vi "UPRcontroller_v00_basedonlsmv66.vi"() -> ()   [LabVIEW 2015] (continued)
                                tunnel: [w4658 _] -> w4656
                                frame #0 {
                                n1663 = call "waveformparamsv2.vi"("command"="get") -> ("Params out"=w4661:T17)  [unwired: 4 in, 2 out]
                                n1664 = Unbundle By Name(w4661) -> ("DO parameters"=w4662:T20)
                                n1665 = Index Array(array=w4662, index=w4659) -> (element=w4658:T21)
                                }
                                frame #1 {
                                w4676 = 0.0 ("padding value")
                                n1666 = call "2pparameters.vi"("command"="get") -> ("params out"=w4674:T12)  [unwired: 1 in]
                                n1667 = Unbundle By Name(w4674) -> ("srate"=w4672:sgl, "Pel"=w4673:sgl)
                                n1668 = To Double Precision Float(number=w4672) -> (double precision float=w4670:dbl)
                                n1669 = To Double Precision Float(number=w4672) -> (double precision float=w4671:dbl)
                                n1670 = To Double Precision Float(number=w4673) -> (double precision float=w4666:dbl)
                                n1671 = Divide(x=1.0 ("Digital DC (%)"), y=w4666) -> (x/y=w4665:dbl)
                                n1672 = Multiply(x=100.0, y=w4665) -> (x*y=w4664:dbl)
                                n1673 = Divide(x=w4671, y=w4666) -> (x/y=w4669:dbl)
                                n1674 = call "replace DO wf param.vi"("Digital Freq (Hz)"=w4669, "Digital DC (%)"=w4664, "Digital phase"=w4676, "Sampling frequency (Hz)"=w4670, "Digital time offset (s)"=w4676, "index of DO wave"=w4668, "padding value"=w4676, "matlab wave file"=path "LT" ("matlab wave number")) -> ()  [unwired: 3 in]
                                }
                                }
                                }
                                }
                                n1675 = Build Array(w4652) -> (w4651:T20)
                                }
                                }
                                }
                                frame #9 {
                                n1676 = Build Array(w4681, w4680) -> (w4683:bool[])
                                n1677 = Boolean Array To Number(Boolean array=w4683) -> (number=w4682:u32)
                                n1678 = case shown="0" w4682 {
                                tunnel: w4679 -> [_ w4735 _ w4739]
                                tunnel: [_ w4730 _ w4736] -> w4678
                                frame 1 {
                                n1679 = call "2pparameters.vi"("command"="get") -> ("params out"=w4690:T12)  [unwired: 1 in]
                                n1680 = Unbundle By Name(w4690) -> ("wavdet"=w4691:bool, "Pel"=w4693:sgl, "refwfsize"=w4694:dbl, "Pel"=w4692:sgl)
                                n1681 = call "waveformsDObuffer.vi"("command"="get") -> ("DO wf out"=w4686:digitalwaveform[])  [unwired: 1 in]
                                n1682 = case shown="True" w4691 {
                                tunnel: [w4698 w4711] -> w4688
                                tunnel: w4692 -> [w4707 w4726]
                                tunnel: w4693 -> [w4697 w4717]
                                tunnel: w4694 -> [_ w4723]
                                frame False {
                                w4701 = u16 0 items=["unsigned binary", "offset binary", "2's complement"] ("data format (offset binary)")
                                n1683 = Initialize Array(sgl 0.0, w4697) -> (w4704:sgl[])
                                n1684 = Replace Array Subset(array=w4704, new element=sgl 1.0, index=0) -> (w4702:sgl[])
                                n1685 = Reciprocal(x=w4707) -> (1/x=w4708:sgl)
                                n1686 = Bundle By Name("Y"=w4702, "dt"=w4708) -> (w4699:waveform(sgl))  [unwired: 1 in]
                                n1687 = call-poly <vilib>:"Analog to Digital.vi"("data format (offset binary)"=w4701, "compress digital (T)"=TRUE, "full-scale range (pk-pk)"=1.0, "resolution (16 bit)"=1, "analog waveform"=w4699) -> ("digital waveform"=w4698:digitalwaveform)  [unwired: 3 in, 3 out]
                                }
                                frame True {
                                w4714 = u16 0 items=["unsigned binary", "offset binary", "2's complement"] ("data format (offset binary)")
                                n1688 = To Double Precision Float(number=w4717) -> (double precision float=w4724:dbl)
                                n1689 = Initialize Array(sgl 0.0, w4717) -> (w4719:sgl[])
                                n1690 = Divide(x=w4723, y=w4724) -> (x/y=w4721:dbl)
                                n1691 = Round Toward +Infinity(x=w4721) -> (ceil(x): smallest int >= x=w4722:dbl)
                                n1692 = Replace Array Subset(array=w4719, new element=sgl 1.0, index=0) -> (w4716:sgl[])
                                n1693 = for {
                                N: w4722 -> [_]
                                tunnel: w4716 -> [w4728]
                                tunnel: [w4728] -> w4725 mode=concatenating
                                }
                                n1694 = Reciprocal(x=w4726) -> (1/x=w4727:sgl)
                                n1695 = Bundle By Name("Y"=w4725, "dt"=w4727) -> (w4712:waveform(sgl))  [unwired: 1 in]
                                n1696 = call-poly <vilib>:"Analog to Digital.vi"("data format (offset binary)"=w4714, "compress digital (T)"=TRUE, "full-scale range (pk-pk)"=1.0, "resolution (16 bit)"=1, "analog waveform"=w4712) -> ("digital waveform"=w4711:digitalwaveform)  [unwired: 3 in, 3 out]
                                }
                                }
                                n1697 = Build Array (concatenate)(w4686, w4688) -> (w4684:digitalwaveform[])
                                n1698 = call "waveformsDObuffer.vi"("DO wf in"=w4684, "command"="set") -> ()  [unwired: 1 out]
                                }
                                frame 2 {
                                n1699 = call "waveformsDObuffer.vi"("command"="get") -> ("DO wf out"=w4732:digitalwaveform[])  [unwired: 1 in]
                                n1700 = Delete From Array(array=w4732, length=1, index=w4735) -> (deleted portion=w4730:digitalwaveform[], array with subset deleted=w4729:digitalwaveform[])
                                n1701 = call "waveformsDObuffer.vi"("DO wf in"=w4729, "command"="set") -> ()  [unwired: 1 out]
                                }
                                frame 3, Default {
                                }
                                frame 0 {
                                n1702 = local read "Measurement"() -> (w4738:T4)
                                n1703 = To Unsigned Long Integer(number=w4738) -> (unsigned 32bit integer=w4737:u32)
                                n1704 = case shown="5..7" w4737 {
                                tunnel: w4739 -> [_ w4742]
                                tunnel: [_ w4741] -> w4736
                                frame 0..4, Default {
                                }
                                frame 5..7 {
                                n1705 = call "2pparameters.vi"("command"="get") -> ("params out"=w4749:T12)  [unwired: 1 in]
                                n1706 = Unbundle By Name(w4749) -> ("wavdet"=w4750:bool, "Pel"=w4752:sgl, "refwfsize"=w4753:dbl, "srateAODO"=w4751:sgl)
                                n1707 = call "waveformsDObuffer.vi"("command"="get") -> ("DO wf out"=w4743:digitalwaveform[])  [unwired: 1 in]
                                n1708 = Index Array(array=w4743, index=w4742) -> (element=w4744:digitalwaveform)
                                n1709 = case shown="True" w4750 {
                                tunnel: [w4757 w4770] -> w4747
                                tunnel: w4751 -> [w4766 w4785]
                                tunnel: w4752 -> [w4756 w4776]
                                tunnel: w4753 -> [_ w4782]
                                frame False {
                                w4760 = u16 0 items=["unsigned binary", "offset binary", "2's complement"] ("data format (offset binary)")
                                n1710 = Initialize Array(sgl 0.0, w4756) -> (w4763:sgl[])
                                n1711 = Replace Array Subset(array=w4763, new element=sgl 1.0, index=0) -> (w4761:sgl[])
                                n1712 = Reciprocal(x=w4766) -> (1/x=w4767:sgl)
                                n1713 = Bundle By Name("Y"=w4761, "dt"=w4767) -> (w4758:waveform(sgl))  [unwired: 1 in]
                                n1714 = call-poly <vilib>:"Analog to Digital.vi"("data format (offset binary)"=w4760, "compress digital (T)"=TRUE, "full-scale range (pk-pk)"=1.0, "resolution (16 bit)"=1, "analog waveform"=w4758) -> ("digital waveform"=w4757:digitalwaveform)  [unwired: 3 in, 3 out]
                                }
                                frame True {
                                w4773 = u16 0 items=["unsigned binary", "offset binary", "2's complement"] ("data format (offset binary)")
                                n1715 = To Double Precision Float(number=w4776) -> (double precision float=w4783:dbl)
                                n1716 = Initialize Array(sgl 0.0, w4776) -> (w4778:sgl[])
                                n1717 = Divide(x=w4782, y=w4783) -> (x/y=w4780:dbl)
                                n1718 = Round Toward +Infinity(x=w4780) -> (ceil(x): smallest int >= x=w4781:dbl)
                                n1719 = Replace Array Subset(array=w4778, new element=sgl 1.0, index=0) -> (w4775:sgl[])
                                n1720 = for {
                                N: w4781 -> [_]
                                tunnel: w4775 -> [w4787]
                                tunnel: [w4787] -> w4784 mode=concatenating
                                }
                                n1721 = Reciprocal(x=w4785) -> (1/x=w4786:sgl)
                                n1722 = Bundle By Name("Y"=w4784, "dt"=w4786) -> (w4771:waveform(sgl))  [unwired: 1 in]
                                n1723 = call-poly <vilib>:"Analog to Digital.vi"("data format (offset binary)"=w4773, "compress digital (T)"=TRUE, "full-scale range (pk-pk)"=1.0, "resolution (16 bit)"=1, "analog waveform"=w4771) -> ("digital waveform"=w4770:digitalwaveform)  [unwired: 3 in, 3 out]
                                }
                                }
                                n1724 = Build Array(w4744) -> (w4741:digitalwaveform[])
                                n1725 = Replace Array Subset(array=w4743, new element=w4747, index=w4742) -> (w4740:digitalwaveform[])
                                n1726 = call "waveformsDObuffer.vi"("DO wf in"=w4740, "command"="set") -> ()  [unwired: 1 out]
                                }
                                }
                                }
                                }
                                }
                                frame #10 {
                                # "Source of crashing?"
                                n1727 = local read "Meastab"() -> (w4801:enum32{"X-Y Image", "Linescan", "Timetrace"})
                                n1728 = property on="refwf" class="Ring (strict)"() -> ("RingText.Text"=w4798:string)  [unwired: 2 in, 2 out]
                                n1729 = case shown="\"Timetrace\"" w4801 {
                                tunnel: [w4803 w4804] -> w4802
                                frame "X-Y Image", Default {
                                n1730 = local read "Sampling rate"() -> (w4803:dbl)
                                }
                                frame "Timetrace" {
                                n1731 = local read "srateAODOtt"() -> (w4804:dbl)
                                }
                                }
                                n1732 = call "waveformsAObuffer.vi"("command"="get") -> ("AO wf out"=w4791:waveform(dbl)[])  [unwired: 1 in]
                                n1733 = local read "wavdet"() -> (w4799:bool)
                                n1734 = call "waveformsDObuffer.vi"("command"="get") -> ("DO wf out"=w4795:digitalwaveform[])  [unwired: 1 in]
                                n1735 = call "correctwaveformsizetemp.vi"("new sampling frequency (Hz)"=w4802, "start"=TRUE, "reference waveforms to"=w4798, "Analog waveforms in"=w4791, "stop"=FALSE, "Digital waveforms in"=w4795) -> ("analog wf out"=w4797:waveform(dbl)[], "Digital wf out"=w4790:digitalwaveform[], "measpoints"=w4800:i32)
                                n1736 = call "waveformsDObuffer.vi"("DO wf in"=w4790, "command"="set") -> ()  [unwired: 1 out]
                                n1737 = call "waveformsAObuffer.vi"("AO wf in"=w4797, "command"="set") -> ()  [unwired: 1 out]
                                n1738 = case shown="True" w4799 {
                                tunnel: w4800 -> [_ w4807]
                                tunnel: w4790 -> [_ w4805]
                                frame False {
                                }
                                frame True {
                                n1739 = local write "# of frames"(w4807) -> ()
                                n1740 = call "GetNumCamFramesv2.vi"("Digital Waveform Graph"=w4805) -> ("Numeric"=w4806:i32)  [unwired: 10 in]
                                n1741 = local write "Total Camera Frames"(w4806) -> ()
                                }
                                }
                                }
                                }
                              }
                              frame #7 {
                                # "Disabled for conversion to 64 bit"
                                # "lifetime related stuff"
                                n1742 = disable-structure shown="Disabled" {
                                frame Disabled {
                                n1743 = local read "Measurement"() -> (w4809:T4)
                                n1744 = case shown="\"Lifetime (scan)\"" w4809 {
                                frame "X-Y-t movie", Default {
                                }
                                frame "Lifetime (scan)" {
                                # "total acquisition time"
                                n1745 = call "2pparameters.vi"("command"="get") -> ("params out"=w4817:T12)  [unwired: 1 in]
                                n1746 = Unbundle By Name(w4817) -> ("measpoints"=w4811:i32, "srateAODO"=w4832:sgl)
                                n1747 = Divide(x=w4811, y=w4832) -> (x/y=w4810:sgl)
                                n1748 = local read "min phot"() -> (w4827:u32)
                                n1749 = local read "expected c/s"() -> (w4828:dbl)
                                n1750 = Multiply(x=w4810, y=1000.0) -> (x*y=w4820:dbl)
                                n1751 = local read "Ch1 ZeroX"() -> (w4825:i32)
                                n1752 = local read "truncate"() -> (w4826:u32)
                                n1753 = To Long Integer(number=w4820) -> (32bit integer=w4829:i32)
                                n1754 = To Long Integer(number=w4828) -> (32bit integer=w4830:i32)
                                n1755 = local read "Number of Bins"() -> (w4821:u32)
                                n1756 = local read "Ch1 Level"() -> (w4823:i32)
                                n1757 = local read "Ch0 ZeroX"() -> (w4824:i32)
                                n1758 = local write "Acquisition time"(w4829) -> ()
                                n1759 = local read "Ch0 Level"() -> (w4822:i32)
                                n1760 = call "lifetimeparameters.vi"("command"="get") -> ("Params out"=w4815:T22)  [unwired: 1 in]
                                n1761 = Add(x=100, y=w4829) -> (x+y=w4819:i32)
                                n1762 = Bundle By Name(cluster=w4815, "acq time"=w4819, "acq rate"=w4830, "# bins"=w4821, "Ch0 Level"=w4822, "Ch1 Level"=w4823, "Ch0 ZeroX"=w4824, "Ch1 ZeroX"=w4825, "min photons"=w4827, "truncate"=w4826) -> (w4814:T22)
                                n1763 = local write "Acquisition rate"(w4830) -> ()
                                n1764 = call "lifetimeparameters.vi"("Params in"=w4814, "command"="set") -> ()  [unwired: 1 out]
                                }
                                }
                                }
                                frame Enabled {
                                }
                                }
                                n1765 = local write "64bit disabled"(TRUE ("64bit disabled")) -> ()
                              }
                              frame #8 {
                                # "setting timeout and sample mode"
                                n1766 = call "2pparameters.vi"("command"="get") -> ("params out"=w4843:T12)  [unwired: 1 in]
                                n1767 = Unbundle By Name(w4843) -> ("refreshbuffer"=w4841:i32, "srate"=w4842:sgl)
                                n1768 = local read "wavdet"() -> (w4833:bool)
                                n1769 = To Double Precision Float(number=w4842) -> (double precision float=w4845:dbl)
                                n1770 = To Double Precision Float(number=w4841) -> (double precision float=w4836:dbl)
                                n1771 = case shown="False" w4833 {
                                tunnel: [w4850 w4851] -> w4835
                                frame False {
                                w4850 = 10123 items=["Finite Samples"=10178, "Continuous Samples"=10123, "Hardware Timed Single Point"=12522] ("sample mode")
                                }
                                frame True {
                                w4851 = 10123 items=["Finite Samples"=10178, "Continuous Samples"=10123, "Hardware Timed Single Point"=12522] ("sample mode")
                                }
                                }
                                n1772 = Divide(x=w4836, y=w4845) -> (x/y=w4849:dbl)
                                n1773 = Multiply(x=w4849, y=2.0) -> (x*y=w4846:dbl)
                                n1774 = Max & Min(x=w4846, y=10.0) -> (max(x,y)=w4837:dbl)  [unwired: 1 out]
                                n1775 = call "2pparameters.vi"("command"="get") -> ("params out"=w4840:T12)  [unwired: 1 in]
                                n1776 = Bundle By Name(cluster=w4840, "timeout"=w4837, "sample mode"=w4835) -> (w4838:T12)
                                n1777 = call "2pparameters.vi"("Params in"=w4838, "command"="set") -> ()  [unwired: 1 out]
                              }
                            }
                          }
                          frame #1 {
                            # "waveform prepped in prep AO img"
                            # "Disabled for conversion to 64 bit"
                            # "start preparing the tasks"
                            n1778 = call "prepAO_img.vi"() -> ("Terminal Name with Device Prefix"=w4853:tag)
                            n1779 = call "prepDO_img.vi"() -> ()  [unwired: 2 in]
                            n1780 = call "prepAI_img.vi"("triggersource"=w4853) -> ()  [unwired: 2 in]
                            n1781 = call "prepCI_img.vi"("ArmStart.DigEdge.Src"=w4853) -> ()  [unwired: 1 in]
                            n1782 = disable-structure shown="Disabled" {
                              frame Disabled {
                                n1783 = local read "Measurement"() -> (w4854:T4)
                                n1784 = case shown="\"Lifetime (contour)\"" w4854 {
                                frame "X-Y-t movie", Default {
                                }
                                frame "Lifetime (contour)" {
                                n1785 = stacked-sequence {
                                frame #0 {
                                n1786 = call "PH-temp.vi"("String"="clear" ("command")) -> ()  [unwired: 2 in, 2 out]
                                n1787 = call "PH-temp-raw.vi"("command"="empty") -> ()  [unwired: 1 in, 1 out]
                                }
                                frame #1 {
                                n1788 = call "calib.vi"() -> ()  [unwired: 1 in]
                                }
                                frame #2 {
                                n1789 = call "setup.vi"() -> ()  [unwired: 1 in]
                                }
                                }
                                }
                                }
                              }
                              frame Enabled {
                              }
                            }
                            n1790 = local write "64bit disabled"(TRUE ("64bit disabled")) -> ()
                          }
                          frame #2 {
                            # "prepares files for saving"
                            n1791 = local read "save\ndata"() -> (w4857:bool)
                            n1792 = case shown="True" w4857 {
                              tunnel: w4858 -> [_ w4862]
                              frame False {
                              }
                              frame True {
                                n1793 = local read "filename prefix"() -> (w4860:string)
                                n1794 = local read "data dir"() -> (w4861:path)
                                n1795 = call "preparebinaryfiles.vi"("filename prefix"=w4860, "data dir"=w4861, "timestamp"=w4862) -> ("full-filename"=w4859:string)  [unwired: 1 in]
                                n1796 = local write "full-filename"(w4859) -> ()
                              }
                            }
                            n1797 = call "preptempbuffers_tt.vi"() -> ()  [unwired: 12 in]
                          }
                          frame #3 {
                            n1798 = local read "wavdet"() -> (w4863:bool)
                            n1799 = case shown="False" w4863 {
                              frame False {
                                n1800 = disable-structure shown="Disabled" {
                                frame Disabled {
                                n1801 = call "2pparameters.vi"("command"="get") -> ("params out"=w4866:T12)  [unwired: 1 in]
                                n1802 = Unbundle By Name(w4866) -> ("autoshutter"=w4867:bool, "aAS"=w4864:u32[])
                                n1803 = case shown="True" w4867 {
                                tunnel: w4864 -> [_ w4868]
                                frame False {
                                }
                                frame True {
                                n1804 = call "shuttercontrol_multi.vi"("Autoshutter Chans"=w4868, "command"="open") -> ()  [unwired: 1 in, 1 out]
                                }
                                }
                                }
                                frame Enabled {
                                }
                                }
                              }
                              frame True {
                              }
                            }
                          }
                          frame #4 {
                            # "start trigger comes from AO, so  start everything and then start AO"
                            n1805 = flat-sequence {
                              frame #0 {
                                # "Disabled for conversion to 64 bit"
                                n1806 = disable-structure shown="Disabled" {
                                frame Disabled {
                                n1807 = local read "Measurement"() -> (w4871:T4)
                                n1808 = case shown="\"Lifetime (contour)\"" w4871 {
                                frame "X-Y-t movie", Default {
                                }
                                frame "Lifetime (contour)" {
                                n1809 = call "runLT_img.vi"() -> ()  [unwired: 1 in]
                                }
                                }
                                }
                                frame Enabled {
                                }
                                }
                                n1810 = local write "64bit disabled"(TRUE ("64bit disabled")) -> ()
                              }
                              frame #1 {
                                n1811 = call "runAI_img.vi"() -> ()  [unwired: 12 in]
                                n1812 = call "runCI.vi"() -> ()  [unwired: 12 in]
                                n1813 = call "runDO_img.vi"() -> ()  [unwired: 12 in]
                              }
                              frame #2 {
                                n1814 = call "runAO_img.vi"() -> ()  [unwired: 12 in]
                              }
                            }
                          }
                          frame #5 {
                            # "Disabled for conversion to 64 bit"
                            n1815 = while {
                              i -> [w4897]
                              stop <- w4895 stop-if-true
                              n1816 = local read "Stop"() -> (w4905:bool)
                              n1817 = local read "Exit"() -> (w4904:bool)
                              n1818 = Or(x=w4905, y=w4904) -> (x .or. y?=w4903:bool)
                              n1819 = case shown="False" w4903 {
                                frame False {
                                n1820 = stacked-sequence {
                                frame #0 {
                                n1821 = call "collectAI_tt_V2.vi"() -> ()  [unwired: 4 in]
                                n1822 = call "collectCI_tt.vi"() -> ("size(s)"=w4912:i32)  [unwired: 3 in]
                                n1823 = local write "scol"(w4912) -> ()
                                }
                                frame #1 {
                                n1824 = local read "Live"() -> (w4913:bool)
                                n1825 = case shown="True" w4913 {
                                frame False {
                                }
                                frame True {
                                n1826 = local read "graph1list"() -> (w4920:u16)
                                n1827 = local read "graph2list"() -> (w4919:u16)
                                n1828 = To Unsigned Word Integer(number=w4920) -> (unsigned 16bit integer=w4918:u16)
                                n1829 = To Unsigned Word Integer(number=w4919) -> (unsigned 16bit integer=w4917:u16)
                                n1830 = call "dattotrace.vi"("graph2list"=w4917, "Current Average"=sgl 1.0, "graph1list"=w4918) -> ("trace2array out"=w4915:sgl[], "trace1array out"=w4926:sgl[])
                                n1831 = local read "bin"() -> (w4927:dbl)
                                n1832 = script code="data=reshape(datain,[bin length(datain)./bin]);\ndataout=mean(data,1);\ndata2=reshape(datain2,[bin length(datain2)./bin]);\ndataout2=mean(data2,1);"("bin"=w4927, "datain"=w4926, "datain2"=w4915) -> ("dataout"=w4925:dbl[], "dataout2"=w4914:dbl[])  [unwired: 1 in, 1 out]
                                n1833 = Array Size(array=w4914) -> (size(s)=w4928:i32)
                                n1834 = Divide(x=w4928, y=2) -> (x/y=w4930:dbl)
                                n1835 = Round To Nearest(number=w4930) -> (nearest integer value=w4932:dbl)
                                n1836 = Array Size(array=w4925) -> (size(s)=w4937:i32)
                                n1837 = Delete From Array(array=w4914, length=w4932, index=0) -> (deleted portion=w4923:dbl[], array with subset deleted=w4924:dbl[])
                                n1838 = Divide(x=w4937, y=2) -> (x/y=w4935:dbl)
                                n1839 = Round To Nearest(number=w4935) -> (nearest integer value=w4933:dbl)
                                n1840 = Delete From Array(array=w4925, length=w4933, index=0) -> (deleted portion=w4922:dbl[], array with subset deleted=w4921:dbl[])
                                n1841 = local write "graph2"(w4921) -> ()
                                n1842 = local write "graph1"(w4922) -> ()
                                n1843 = local write "graph3"(w4923) -> ()
                                n1844 = local write "graph4"(w4924) -> ()
                                }
                                }
                                }
                                frame #2 {
                                n1845 = local read "save\ndata"() -> (w4938:bool)
                                n1846 = case shown="True" w4938 {
                                frame False {
                                }
                                frame True {
                                n1847 = call "savebinaryfiles.vi"() -> ()  [unwired: 1 in]
                                }
                                }
                                }
                                }
                                }
                                frame True {
                                }
                              }
                              n1848 = Increment(x=w4897) -> (x+1=w4896:i32)
                              n1849 = local write "points recorded"(w4896) -> ()
                              n1850 = local read "continuous"() -> (w4900:bool)
                              n1851 = case shown="False" w4900 {
                                tunnel: w4896 -> [w4910 _]
                                tunnel: [w4909 FALSE] -> w4898
                                frame False {
                                n1852 = call "2pparameters.vi"("command"="get") -> ("params out"=w4907:T12)  [unwired: 1 in]
                                n1853 = Unbundle By Name(w4907) -> ("tt_cycles"=w4906:i32)
                                n1854 = Greater Or Equal?(x=w4910, y=w4906) -> (x >= y?=w4909:bool)
                                }
                                frame True {
                                }
                              }
                              n1855 = local read "Stop"() -> (w4902:bool)
                              n1856 = local read "Exit"() -> (w4901:bool)
                              n1857 = Or(x=w4902, y=w4901) -> (x .or. y?=w4899:bool)
                              n1858 = Or(x=w4899, y=w4898) -> (x .or. y?=w4895:bool)
                            }
                            n1859 = disable-structure shown="Disabled" {
                              disable-tunnel: w4873 -> [w4874 _]
                              frame Disabled {
                                w4877 = u16 0 items=["Stream to disk", "Post process", "real time process"] ("Ring")
                                n1860 = local read "T3R Data processing"() -> (w4876:u16)
                                n1861 = Equal?(x=w4876, y=w4877) -> (x = y?=w4875:bool)
                                n1862 = local read "save\ndata"() -> (w4879:bool)
                                n1863 = local read "Measurement"() -> (w4880:T4)
                                n1864 = And(x=w4879, y=w4875) -> (x .and. y?=w4878:bool)
                                n1865 = case shown="\"Lifetime (contour)\"" w4880 {
                                tunnel: w4874 -> [_ w4884]
                                tunnel: w4878 -> [_ w4882]
                                frame "X-Y-t movie", Default {
                                }
                                frame "Lifetime (contour)" {
                                n1866 = case shown="True" w4882 {
                                selector: w4882 -> [w4885 w4890]
                                tunnel: w4884 -> [_ w4888]
                                tunnel: [path "" ("appended path") w4891] -> w4883
                                tunnel: [w4885 w4890] -> w4881
                                frame False {
                                }
                                frame True {
                                n1867 = local read "filename prefix"() -> (w4889:string)
                                n1868 = local read "data dir"() -> (w4892:path)
                                n1869 = call "generatedatafilename.vi"("timestamp"=w4888, "filename prefix in"=w4889) -> ("full-filename"=w4887:string)
                                n1870 = Concatenate Strings(w4887, ".lvpt3contour" ("string")) -> (w4894:string)
                                n1871 = Build Path(base path=w4892, name or relative path=w4894) -> (appended path=w4891:path)
                                }
                                }
                                n1872 = call "collectLT_res_v1.vi"("stream?"=w4881, "data file"=w4883) -> ()  [unwired: 2 out]
                                }
                                }
                              }
                              frame Enabled {
                              }
                            }
                            n1873 = local write "64bit disabled"(TRUE ("64bit disabled")) -> ()
                          }
                          frame #6 {
                            # "Disabled for conversion to 64 bit"
                            n1874 = local read "Measurement"() -> (w4941:T4)
                            n1875 = disable-structure shown="Disabled" {
                              disable-tunnel: w4941 -> [w4943 _]
                              disable-tunnel: w4940 -> [w4942 _]
                              frame Disabled {
                                n1876 = case shown="\"Lifetime (contour)\"" w4943 {
                                tunnel: w4942 -> [_ w4944]
                                frame "X-Y-t movie", Default {
                                }
                                frame "Lifetime (contour)" {
                                n1877 = stacked-sequence {
                                tunnel: w4944 -> [_ w4945]
                                frame #0 {
                                n1878 = flat-sequence {
                                frame #0 {
                                n1879 = call "stoperaseLT_img.vi"() -> ()  [unwired: 1 in]
                                }
                                }
                                }
                                frame #1 {
                                w4948 = u16 0 items=["Stream to disk", "Post process", "real time process"] ("Ring")
                                n1880 = local read "T3R Data processing"() -> (w4947:u16)
                                n1881 = local read "save\ndata"() -> (w4950:bool)
                                n1882 = Equal?(x=w4947, y=w4948) -> (x = y?=w4946:bool)
                                n1883 = Not(x=w4946) -> (.not. x?=w4951:bool)
                                n1884 = And(x=w4950, y=w4951) -> (x .and. y?=w4949:bool)
                                n1885 = case shown="True" w4949 {
                                tunnel: w4945 -> [_ w4952]
                                frame False {
                                }
                                frame True {
                                n1886 = local read "filename prefix"() -> (w4953:string)
                                n1887 = local read "data dir"() -> (w4969:path)
                                n1888 = call "2pparameters.vi"("command"="get") -> ("params out"=w4964:T12)  [unwired: 1 in]
                                n1889 = call "generatedatafilename.vi"("timestamp"=w4952, "filename prefix in"=w4953) -> ("full-filename"=w4954:string)
                                n1890 = Unbundle By Name(w4964) -> ("srate"=w4962:sgl, "Pel"=w4961:sgl, "measpoints"=w4959:i32)
                                n1891 = Concatenate Strings(w4954, ".lvpt3contour" ("string")) -> (w4967:string)
                                n1892 = Build Path(base path=w4969, name or relative path=w4967) -> (appended path=w4966:path)
                                n1893 = To Unsigned Long Integer(number=w4962) -> (unsigned 32bit integer=w4963:u32)
                                n1894 = To Unsigned Long Integer(number=w4961) -> (unsigned 32bit integer=w4960:u32)
                                n1895 = To Unsigned Long Integer(number=w4959) -> (unsigned 32bit integer=w4958:u32)
                                n1896 = call "PH-temp-raw.vi"("command"="get") -> ("array out"=w4957:u32[])  [unwired: 1 in]
                                n1897 = Build Array (concatenate)(w4963, w4960, w4958, w4957) -> (w4956:u32[])
                                n1898 = Open/Create/Replace File(file path (use dialog)=w4966, operation (0:open)=T9."replace or create") -> (refnum out=w4973:refnum<file>, error out=w4972:errorcluster)  [unwired: 4 in, 1 out]
                                n1899 = Write to Binary File(file (use dialog)=w4973, data=w4956, error in=w4972, 5:FALSE ("prepend array or string size? (T)")) -> (refnum out=w4970:refnum<file>, error out=w4971:errorcluster)  [unwired: 2 in, 1 out]
                                n1900 = Close File(refnum=w4970, error in=w4971) -> ()  [unwired: 2 out]
                                }
                                }
                                }
                                }
                                }
                                }
                              }
                              frame Enabled {
                              }
                            }
                            n1901 = local write "64bit disabled"(TRUE ("64bit disabled")) -> ()
                          }
                          frame #7 {
                            n1902 = flat-sequence {
                              frame #0 {
                                n1903 = call "reset AO_DO_v3.vi"() -> ()  [unwired: 12 in]
                              }
                              frame #1 {
                                n1904 = call "stoperaseCI.vi"() -> ()  [unwired: 12 in]
                                n1905 = call "stoperaseDO_img.vi"() -> ()  [unwired: 12 in]
                                n1906 = call "stoperaseAO_img.vi"() -> ()  [unwired: 12 in]
                                n1907 = call "stoperaseAI_img.vi"() -> ()  [unwired: 12 in]
                              }
                            }
                          }
                          frame #8 {
                            n1908 = stacked-sequence {
                              tunnel: w4989 -> [w4992 _ _ _ _ _]
                              tunnel: w4986 -> [w4991 _ _ _ _ _]
                              tunnel: w4987 -> [w4990 _ _ _ _ _]
                              tunnel: w4988 -> [_ w5041 _ _ _ _]
                              tunnel: w4984 -> [_ w5040 w5091 w5214 _ _]
                              tunnel: w4985 -> [_ w5039 w5092 w5213 _ _]
                              tunnel: w4983 -> [_ _ _ w5212 _ _]
                              tunnel: w4982 -> [_ _ _ w5211 _ _]
                              tunnel: w4981 -> [_ _ w5094 _ _ _]
                              tunnel: w4980 -> [_ _ w5093 _ _ _]
                              tunnel: w4979 -> [_ _ w5088 _ _ _]
                              tunnel: w4978 -> [_ _ w5089 _ _ _]
                              tunnel: w4977 -> [_ _ _ w5209 _ _]
                              tunnel: w4976 -> [_ _ _ w5208 _ _]
                              frame #0 {
                                n1909 = case shown="True" w4992 {
                                tunnel: w4991 -> [_ w5014]
                                tunnel: w4990 -> [_ w5013]
                                frame True {
                                n1910 = stacked-sequence {
                                seq-local: [w4993 _ _] -> [_ w5005 w5010]
                                frame #0 {
                                n1911 = call "configuration.vi"("command"="get") -> ("config out"=w4999:T14)  [unwired: 2 in, 1 out]
                                n1912 = Unbundle By Name(w4999) -> ("Voltage to Xgalvo"=w4996:i32)
                                n1913 = call "2pparameters.vi"("command"="get") -> ("params out"=w4997:T12)  [unwired: 1 in]
                                n1914 = in-place {
                                in-place-border: w4996 -> [w5004]
                                in-place-border: [w5001] -> w4993
                                n1915 = in-place-cluster #31(w4997) -> ("aAO"=w5003:u32[])
                                n1916 = call "remove channel from active arrayv2.vi"("line array in"=w5003, "line to remove"=w5004) -> ("line array out"=w5002:u32[], "index"=w5001:i32)  [unwired: 1 out]
                                n1917 = in-place-cluster #31("aAO"=w5002) -> (w4994:T12)
                                }
                                n1918 = call "2pparameters.vi"("Params in"=w4994, "command"="set") -> ()  [unwired: 1 out]
                                }
                                frame #1 {
                                n1919 = call "waveformparamsv2.vi"("command"="rem AO", "index"=w5005) -> ()  [unwired: 3 in, 3 out]
                                }
                                frame #2 {
                                n1920 = call "waveformsAObuffer.vi"("command"="get") -> ("AO wf out"=w5011:waveform(dbl)[])  [unwired: 1 in]
                                n1921 = Delete From Array(array=w5011, length=1, index=w5010) -> (array with subset deleted=w5007:waveform(dbl)[])  [unwired: 1 out]
                                n1922 = call "waveformsAObuffer.vi"("AO wf in"=w5007, "command"="set") -> ()  [unwired: 1 out]
                                }
                                }
                                }
                                frame False {
                                n1923 = stacked-sequence {
                                seq-local: [w5015 _ _] -> [_ w5023 w5034]
                                tunnel: w5014 -> [_ w5022 _]
                                tunnel: w5013 -> [_ _ w5033]
                                frame #0 {
                                n1924 = call "configuration.vi"("command"="get") -> ("config out"=w5020:T14)  [unwired: 2 in, 1 out]
                                n1925 = Unbundle By Name(w5020) -> ("Voltage to Xgalvo"=w5016:i32)
                                n1926 = call "2pparameters.vi"("command"="get") -> ("params out"=w5019:T12)  [unwired: 1 in]
                                n1927 = Unbundle By Name(w5019) -> ("aAO"=w5017:u32[])
                                n1928 = Search 1D Array(1D array=w5017, element=w5016) -> (index of element=w5015:i32)  [unwired: 1 in]
                                }
                                frame #1 {
                                n1929 = call "waveformparamsv2.vi"("command"="get") -> ("Params out"=w5026:T17)  [unwired: 4 in, 2 out]
                                n1930 = in-place {
                                in-place-border: w5023 -> [w5030]
                                in-place-border: w5022 -> [w5029]
                                n1931 = in-place-cluster #32(w5026) -> ("AO parameters"=w5031:T18)
                                n1932 = in-place {
                                in-place-border: w5029 -> [w5032]
                                n1933 = in-place-array #33(w5031, w5030) -> ()  [unwired: 1 out]
                                n1934 = in-place-array #33(w5032) -> (w5028:T18)  [unwired: 1 out]
                                }
                                n1935 = in-place-cluster #32("AO parameters"=w5028) -> (w5024:T17)
                                }
                                n1936 = call "waveformparamsv2.vi"("command"="set", "Params in"=w5024) -> ()  [unwired: 3 in, 3 out]
                                }
                                frame #2 {
                                n1937 = call "waveformsAObuffer.vi"("command"="get") -> ("AO wf out"=w5037:waveform(dbl)[])  [unwired: 1 in]
                                n1938 = Replace Array Subset(array=w5037, new element=w5033, index=w5034) -> (w5035:waveform(dbl)[])
                                n1939 = call "waveformsAObuffer.vi"("AO wf in"=w5035, "command"="set") -> ()  [unwired: 1 out]
                                }
                                }
                                }
                                }
                              }
                              frame #1 {
                                n1940 = case shown="True" w5041 {
                                tunnel: w5040 -> [_ w5063]
                                tunnel: w5039 -> [_ w5062]
                                frame True {
                                n1941 = stacked-sequence {
                                seq-local: [w5042 _ _] -> [_ w5054 w5059]
                                frame #0 {
                                n1942 = call "configuration.vi"("command"="get") -> ("config out"=w5048:T14)  [unwired: 2 in, 1 out]
                                n1943 = Unbundle By Name(w5048) -> ("Voltage to Ygalvo"=w5045:i32)
                                n1944 = call "2pparameters.vi"("command"="get") -> ("params out"=w5046:T12)  [unwired: 1 in]
                                n1945 = in-place {
                                in-place-border: w5045 -> [w5053]
                                in-place-border: [w5050] -> w5042
                                n1946 = in-place-cluster #34(w5046) -> ("aAO"=w5052:u32[])
                                n1947 = call "remove channel from active arrayv2.vi"("line array in"=w5052, "line to remove"=w5053) -> ("line array out"=w5051:u32[], "index"=w5050:i32)  [unwired: 1 out]
                                n1948 = in-place-cluster #34("aAO"=w5051) -> (w5043:T12)
                                }
                                n1949 = call "2pparameters.vi"("Params in"=w5043, "command"="set") -> ()  [unwired: 1 out]
                                }
                                frame #1 {
                                n1950 = call "waveformparamsv2.vi"("command"="rem AO", "index"=w5054) -> ()  [unwired: 3 in, 3 out]
                                }
                                frame #2 {
                                n1951 = call "waveformsAObuffer.vi"("command"="get") -> ("AO wf out"=w5060:waveform(dbl)[])  [unwired: 1 in]
                                n1952 = Delete From Array(array=w5060, length=1, index=w5059) -> (array with subset deleted=w5056:waveform(dbl)[])  [unwired: 1 out]
                                n1953 = call "waveformsAObuffer.vi"("AO wf in"=w5056, "command"="set") -> ()  [unwired: 1 out]
                                }
                                }
                                }
                                frame False {
                                n1954 = stacked-sequence {
                                seq-local: [w5064 _ _] -> [_ w5072 w5083]
                                tunnel: w5063 -> [_ w5071 _]
                                tunnel: w5062 -> [_ _ w5082]
                                frame #0 {
                                n1955 = call "configuration.vi"("command"="get") -> ("config out"=w5069:T14)  [unwired: 2 in, 1 out]
                                n1956 = Unbundle By Name(w5069) -> ("Voltage to Ygalvo"=w5065:i32)
                                n1957 = call "2pparameters.vi"("command"="get") -> ("params out"=w5068:T12)  [unwired: 1 in]
                                n1958 = Unbundle By Name(w5068) -> ("aAO"=w5066:u32[])
                                n1959 = Search 1D Array(1D array=w5066, element=w5065) -> (index of element=w5064:i32)  [unwired: 1 in]
                                }
                                frame #1 {
                                n1960 = call "waveformparamsv2.vi"("command"="get") -> ("Params out"=w5075:T17)  [unwired: 4 in, 2 out]
                                n1961 = in-place {
                                in-place-border: w5072 -> [w5079]
                                in-place-border: w5071 -> [w5078]
                                n1962 = in-place-cluster #35(w5075) -> ("AO parameters"=w5080:T18)
                                n1963 = in-place {
                                in-place-border: w5078 -> [w5081]
                                n1964 = in-place-array #36(w5080, w5079) -> ()  [unwired: 1 out]
                                n1965 = in-place-array #36(w5081) -> (w5077:T18)  [unwired: 1 out]
                                }
                                n1966 = in-place-cluster #35("AO parameters"=w5077) -> (w5073:T17)
                                }
                                n1967 = call "waveformparamsv2.vi"("command"="set", "Params in"=w5073) -> ()  [unwired: 3 in, 3 out]
                                }
                                frame #2 {
                                n1968 = call "waveformsAObuffer.vi"("command"="get") -> ("AO wf out"=w5086:waveform(dbl)[])  [unwired: 1 in]
                                n1969 = Replace Array Subset(array=w5086, new element=w5082, index=w5083) -> (w5084:waveform(dbl)[])
                                n1970 = call "waveformsAObuffer.vi"("AO wf in"=w5084, "command"="set") -> ()  [unwired: 1 out]
                                }
                                }
                                }
                                }
                              }
                              frame #2 {
                                n1971 = Build Array(w5094, w5093) -> (w5095:bool[])
                                n1972 = Boolean Array To Number(Boolean array=w5095) -> (number=w5090:u32)
                                n1973 = case shown="0" w5090 {
                                tunnel: w5091 -> [_ _ w5155]
                                tunnel: w5092 -> [_ _ w5154]
                                tunnel: w5088 -> [_ w5125 w5152]
                                tunnel: w5089 -> [_ w5124 w5153]
                                frame 1, Default {
                                n1974 = stacked-sequence {
                                seq-local: [w5098 _ _] -> [_ w5110 w5115]
                                frame #0 {
                                # "Remove autoshutter channel from DO list in 2p parameters"
                                n1975 = call "2pparameters.vi"("command"="get") -> ("params out"=w5097:T12)  [unwired: 1 in]
                                n1976 = Unbundle By Name(w5097) -> ("aAS"=w5096:u32[])
                                n1977 = for {
                                tunnel: [w5104] -> w5098 mode=indexing
                                tunnel: w5096 -> [w5102] mode=indexing
                                shift-right: [w5105] -> w5099
                                shift-left: w5097 -> [w5103]
                                n1978 = in-place {
                                in-place-border: w5102 -> [w5109]
                                in-place-border: [w5106] -> w5104
                                n1979 = in-place-cluster #37(w5103) -> ("aDO"=w5108:u32[])
                                n1980 = call "remove channel from active arrayv2.vi"("line array in"=w5108, "line to remove"=w5109) -> ("line array out"=w5107:u32[], "index"=w5106:i32)  [unwired: 1 out]
                                n1981 = in-place-cluster #37("aDO"=w5107) -> (w5105:T12)
                                }
                                }
                                n1982 = call "2pparameters.vi"("Params in"=w5099, "command"="set") -> ()  [unwired: 1 out]
                                }
                                frame #1 {
                                n1983 = for {
                                tunnel: w5110 -> [w5111] mode=indexing
                                n1984 = call "waveformparamsv2.vi"("command"="rem DO", "index"=w5111) -> ()  [unwired: 3 in, 3 out]
                                }
                                }
                                frame #2 {
                                # "sort so it removes the last elements first\nand does not mess up the order"
                                # "Remove waveforms of autoshutter channels from wave forms DO"
                                n1985 = call "waveformsDObuffer.vi"("command"="get") -> ("DO wf out"=w5118:digitalwaveform[])  [unwired: 1 in]
                                n1986 = Sort 1D Array(array=w5115) -> (sorted array=w5114:i32[])
                                n1987 = Reverse 1D Array(array=w5114) -> (reversed array=w5113:i32[])
                                n1988 = for {
                                tunnel: w5113 -> [w5120] mode=indexing
                                shift-right: [w5121] -> w5116
                                shift-left: w5118 -> [w5123]
                                n1989 = Delete From Array(array=w5123, length=1, index=w5120) -> (array with subset deleted=w5121:digitalwaveform[])  [unwired: 1 out]
                                }
                                n1990 = call "waveformsDObuffer.vi"("DO wf in"=w5116, "command"="set") -> ()  [unwired: 1 out]
                                }
                                }
                                }
                                frame 2 {
                                n1991 = stacked-sequence {
                                tunnel: w5125 -> [_ w5139 _]
                                tunnel: w5124 -> [_ _ w5146]
                                frame #0 {
                                # "add autoshutter channels to digital out"
                                n1992 = disable-structure shown="Disabled" {
                                frame Disabled {
                                n1993 = call "configuration.vi"("command"="get") -> ("config out"=w5131:T14)  [unwired: 2 in, 1 out]
                                n1994 = Unbundle By Name(w5131) -> ()  [unwired: 1 out]
                                }
                                frame Enabled {
                                }
                                }
                                n1995 = call "2pparameters.vi"("command"="get") -> ("params out"=w5127:T12)  [unwired: 1 in]
                                n1996 = Unbundle By Name(w5127) -> ("aAS"=w5126:u32[])
                                n1997 = in-place {
                                in-place-border: w5126 -> [w5133]
                                n1998 = in-place-cluster #38(w5127) -> ("aDO"=w5135:u32[])
                                n1999 = for {
                                shift-right: [w5137] -> w5134
                                shift-left: w5135 -> [w5138]
                                tunnel: w5133 -> [w5136] mode=indexing
                                n2000 = call "add channel to active arrayv2.vi"("line array in"=w5138, "line to add"=w5136) -> ("line array out"=w5137:u32[])  [unwired: 2 out]
                                }
                                n2001 = in-place-cluster #38("aDO"=w5134) -> (w5128:T12)
                                }
                                n2002 = call "2pparameters.vi"("Params in"=w5128, "command"="set") -> ()  [unwired: 1 out]
                                }
                                frame #1 {
                                # "Not sure the correct way to add multiple sets of parameters..."
                                # "add autoshutter waveforms to wf parameters v2"
                                n2003 = disable-structure shown="Disabled" {
                                disable-tunnel: w5139 -> [w5141 _]
                                frame Disabled {
                                n2004 = for {
                                tunnel: w5141 -> [w5142] mode=indexing
                                n2005 = call "waveformparamsv2.vi"("command"="add DO", "add DO"=w5142) -> ()  [unwired: 3 in, 3 out]
                                }
                                }
                                frame Enabled {
                                }
                                }
                                n2006 = call "waveformparamsv2.vi"("command"="add DO", "add DO"=w5139) -> ()  [unwired: 3 in, 3 out]
                                }
                                frame #2 {
                                # "add autoshutter waveforms to wave forms DO"
                                n2007 = call "waveformsDObuffer.vi"("command"="get") -> ("DO wf out"=w5147:digitalwaveform[])  [unwired: 1 in]
                                n2008 = for {
                                tunnel: w5146 -> [w5150] mode=indexing
                                shift-right: [w5149] -> w5144
                                shift-left: w5147 -> [w5151]
                                n2009 = Build Array (concatenate)(w5151, w5150) -> (w5149:digitalwaveform[])
                                }
                                n2010 = call "waveformsDObuffer.vi"("DO wf in"=w5144, "command"="set") -> ()  [unwired: 1 out]
                                }
                                }
                                }
                                frame 0 {
                                n2011 = stacked-sequence {
                                seq-local: [w5157 _ _] -> [_ w5165 w5189]
                                tunnel: w5155 -> [_ _ _]
                                tunnel: w5154 -> [_ _ _]
                                tunnel: w5153 -> [_ _ w5188]
                                tunnel: w5152 -> [_ w5164 _]
                                frame #0 {
                                n2012 = call "2pparameters.vi"("command"="get") -> ("params out"=w5160:T12)  [unwired: 1 in]
                                n2013 = Unbundle By Name(w5160) -> ("aDO"=w5158:u32[], "aAS"=w5156:u32[])
                                n2014 = for {
                                tunnel: w5158 -> [w5163]
                                tunnel: [w5162] -> w5157 mode=indexing
                                tunnel: w5156 -> [w5161] mode=indexing
                                n2015 = Search 1D Array(1D array=w5163, element=w5161) -> (index of element=w5162:i32)  [unwired: 1 in]
                                }
                                }
                                frame #1 {
                                n2016 = call "2pparameters.vi"("command"="get") -> ("params out"=w5168:T12)  [unwired: 1 in]
                                n2017 = Unbundle By Name(w5168) -> ("wavdet"=w5166:bool, "autoshutter"=w5167:bool)
                                n2018 = case shown="True" w5167 {
                                tunnel: w5165 -> [_ w5172]
                                tunnel: w5166 -> [_ w5171]
                                tunnel: w5164 -> [_ w5170]
                                frame False {
                                }
                                frame True {
                                n2019 = case shown="False" w5171 {
                                tunnel: w5172 -> [w5174 _]
                                tunnel: w5170 -> [w5173 _]
                                frame False {
                                # "Replace autoshutter channel DO waveforms with those that were generated from autoshutter."
                                n2020 = call "waveformparamsv2.vi"("command"="get") -> ("Params out"=w5177:T17)  [unwired: 4 in, 2 out]
                                n2021 = in-place {
                                in-place-border: w5174 -> [w5181]
                                in-place-border: w5173 -> [w5179]
                                n2022 = in-place-cluster #39(w5177) -> ("DO parameters"=w5182:T20)
                                n2023 = for {
                                tunnel: w5181 -> [w5185] mode=indexing
                                tunnel: w5179 -> [w5183] mode=indexing
                                shift-right: [w5184] -> w5180
                                shift-left: w5182 -> [w5186]
                                n2024 = in-place {
                                in-place-border: w5183 -> [w5187]
                                n2025 = in-place-array #40(w5186, w5185) -> ()  [unwired: 1 out]
                                n2026 = in-place-array #40(w5187) -> (w5184:T20)  [unwired: 1 out]
                                }
                                }
                                n2027 = in-place-cluster #39("DO parameters"=w5180) -> (w5175:T17)
                                }
                                n2028 = call "waveformparamsv2.vi"("command"="set", "Params in"=w5175) -> ()  [unwired: 3 in, 3 out]
                                }
                                frame True {
                                }
                                }
                                }
                                }
                                }
                                frame #2 {
                                n2029 = call "2pparameters.vi"("command"="get") -> ("params out"=w5192:T12)  [unwired: 1 in]
                                n2030 = Unbundle By Name(w5192) -> ("wavdet"=w5190:bool, "autoshutter"=w5191:bool)
                                n2031 = case shown="True" w5191 {
                                tunnel: w5189 -> [_ w5196]
                                tunnel: w5190 -> [_ w5195]
                                tunnel: w5188 -> [_ w5194]
                                frame False {
                                }
                                frame True {
                                n2032 = case shown="False" w5195 {
                                tunnel: w5196 -> [w5198 _]
                                tunnel: w5194 -> [w5197 _]
                                frame False {
                                # "replace autoshutter channels of waveforms DO with autoshutter waveforms"
                                n2033 = call "waveformsDObuffer.vi"("command"="get") -> ("DO wf out"=w5200:digitalwaveform[])  [unwired: 1 in]
                                n2034 = for {
                                tunnel: w5198 -> [w5204] mode=indexing
                                tunnel: w5197 -> [w5203] mode=indexing
                                shift-right: [w5206] -> w5202
                                shift-left: w5200 -> [w5205]
                                n2035 = Replace Array Subset(array=w5205, new element=w5203, index=w5204) -> (w5206:digitalwaveform[])
                                }
                                n2036 = call "waveformsDObuffer.vi"("DO wf in"=w5202, "command"="set") -> ()  [unwired: 1 out]
                                }
                                frame True {
                                }
                                }
                                }
                                }
                                }
                                }
                                }
                                }
                              }
                              frame #3 {
                                n2037 = Build Array(w5209, w5208) -> (w5210:bool[])
                                n2038 = Boolean Array To Number(Boolean array=w5210) -> (number=w5207:u32)
                                n2039 = case shown="2" w5207 {
                                tunnel: w5214 -> [_ _ w5257]
                                tunnel: w5213 -> [_ _ w5256]
                                tunnel: w5212 -> [_ w5236 w5254]
                                tunnel: w5211 -> [_ w5235 w5255]
                                frame 1, Default {
                                n2040 = stacked-sequence {
                                seq-local: [w5215 _ _] -> [_ w5227 w5232]
                                frame #0 {
                                n2041 = call "configuration.vi"("command"="get") -> ("config out"=w5221:T14)  [unwired: 2 in, 1 out]
                                n2042 = Unbundle By Name(w5221) -> ("LT timestamp"=w5218:u32)
                                n2043 = call "2pparameters.vi"("command"="get") -> ("params out"=w5219:T12)  [unwired: 1 in]
                                n2044 = in-place {
                                in-place-border: w5218 -> [w5226]
                                in-place-border: [w5223] -> w5215
                                n2045 = in-place-cluster #41(w5219) -> ("aDO"=w5225:u32[])
                                n2046 = call "remove channel from active arrayv2.vi"("line array in"=w5225, "line to remove"=w5226) -> ("line array out"=w5224:u32[], "index"=w5223:i32)  [unwired: 1 out]
                                n2047 = in-place-cluster #41("aDO"=w5224) -> (w5216:T12)
                                }
